vi "adam-init.vi"(8 "error in (no error)":errorcluster, 10 "baud rate (19200)":u32=19200, 11 "COM Port (COM10)":refnum<visa-resource-name>="COM10") -> (0 "error out":errorcluster, 3 "VISA resource name out":refnum<visa-resource-name>)   [LabVIEW 2021]
uses:
  <vilib>/Instr/_visa.llb/VISA Configure Serial Port (Instr).vi
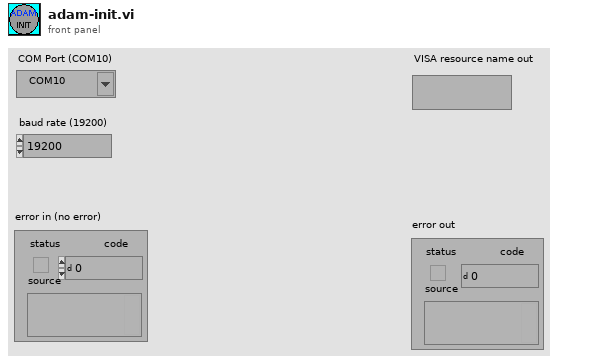
[diagram p1: front panel]
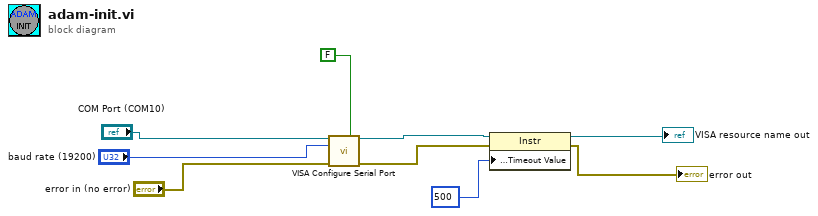
[diagram p0: block diagram]
diagram:
  n1 = call-poly "VISA Configure Serial Port"("VISA resource name"="COM Port (COM10)", "Enable Termination\nChar (T)"=FALSE ("Enable Termination\nChar (T)"), "baud rate (9600)"="baud rate (19200)", "error in (no error)"="error in (no error)") -> ("VISA resource name out"=w3:refnum<visa-resource-name>, "error out"=w4:errorcluster)  [unwired: 10 in]
  n2 = property class="Instr"(reference=w3, error in=w4, "General Settings:Timeout Value"=u32 500) -> (reference out=→"VISA resource name out":refnum<visa-resource-name>, error out=→"error out":errorcluster)
